vi "call_Python_Function.vi"   [LabVIEW 2024]
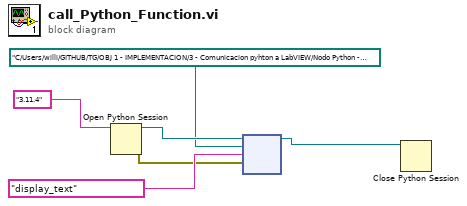
[diagram p0: block diagram]
diagram:
  n1 = Open Python Session(python version="3.11.4" ("Python version")) -> (session out=w5:refnum<k35>, error out=w1:errorcluster)  [unwired: 2 in]
  n2 = node(w5, path "C:/Users/willi/GITHUB/TG/OBJ 1 - IMPLEMENTACION/3 - Comunicacion pyhton a LabVIEW/Nodo Python - Labview native/app.py" ("module path"), "display_text" ("function name"), w1) -> (w4:refnum<k35>)  [unwired: 2 in, 3 out]
  n3 = Close Python Session(session in=w4) -> ()  [unwired: 1 in, 1 out]
